vi "notes_load_xml.vi"(8 "error in":errorcluster, 10 "child node in":refnum<k20>) -> (0 "error out":errorcluster, 2 "child node out":refnum<k20>, 3 "notes":string)   [LabVIEW 2012]
doc: "Loads notes from xml file. Expected format for xml node passed in is:\n\n<Notes>%s</Notes>\n\nMTL 2013 Jan 1"
uses:
  <vilib>/xml/Close Reference(Node).vi
  <vilib>/xml/NI_XML.lvlib
  <resource>/objmgr/DOMUserDefRef.rc
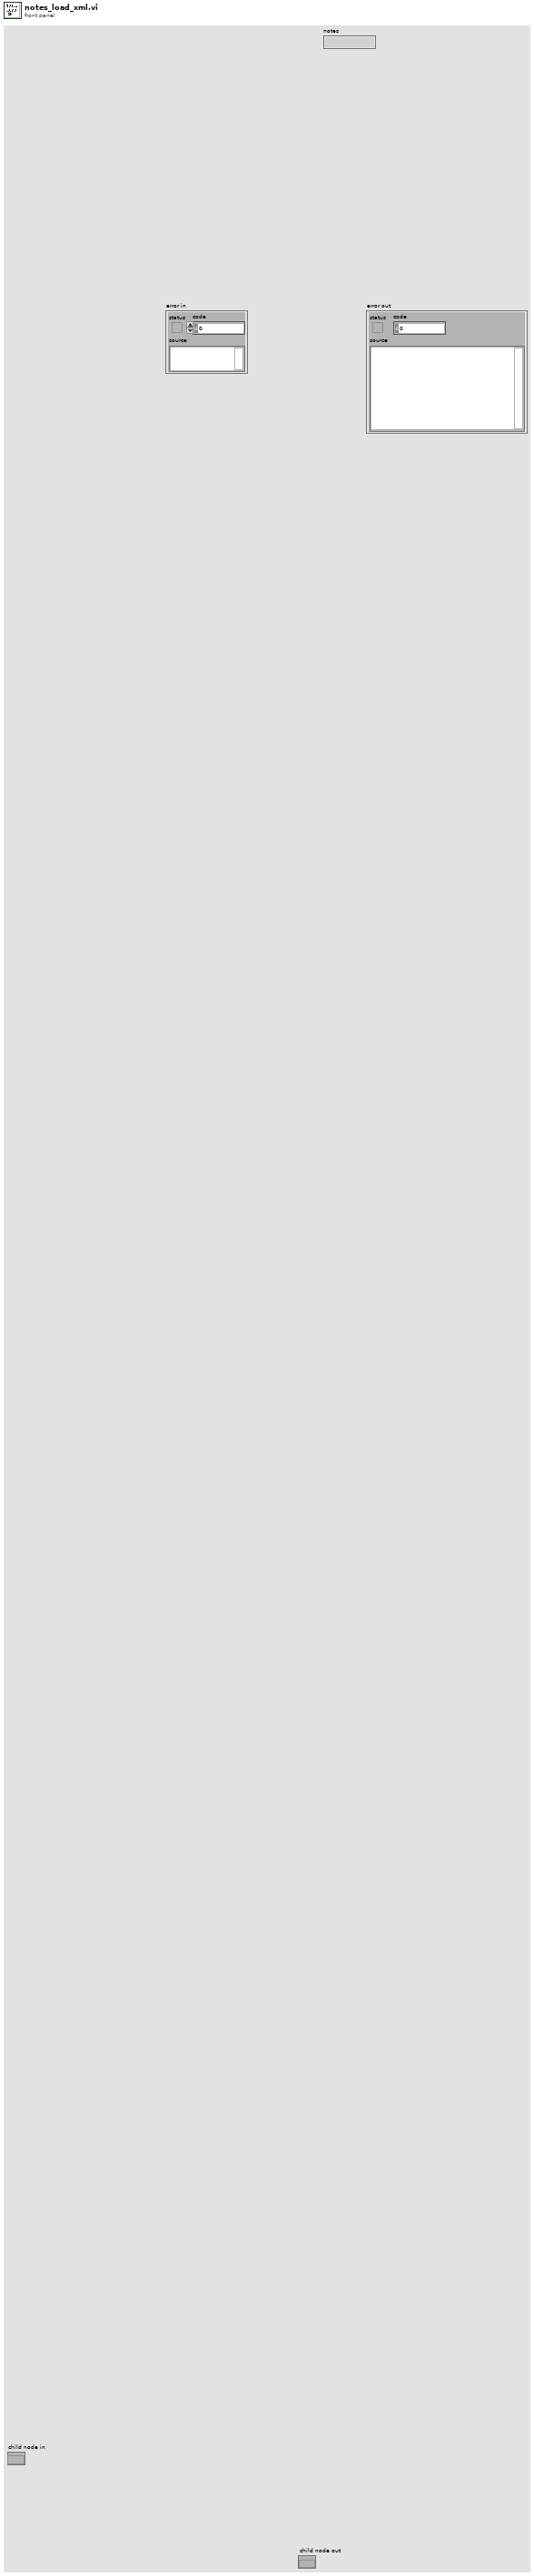
[diagram p1: front panel]
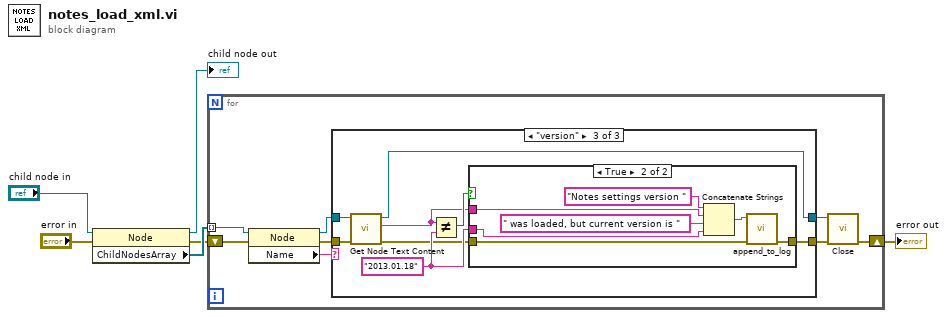
[diagram p0: block diagram]
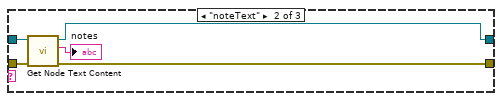
[diagram p3: hidden frame]
diagram:
  n1 = property class="Node"(reference="child node in", error in="error in") -> (reference out=→"child node out":refnum<k20>, error out=w2:errorcluster, "ChildNodesArray"=w4:refnum<k20>[])
  n2 = for {
    tunnel: w4 -> [w14] mode=indexing
    shift-right: [w12] -> w1
    shift-left: w2 -> [w13]
    n3 = property class="Node"(reference=w14, error in=w13) -> (reference out=w11:refnum<k20>, error out=w9:errorcluster, "Name"=w8:string)
    n4 = case shown="\"version\"" w8 {
      tunnel: w11 -> [w16 w18 w28]
      tunnel: [w15 w19 w23] -> w10
      tunnel: w9 -> [w15 w20 w29]
      tunnel: [w16 w17 w22] -> w7
      frame "None", Default {
      }
      frame "noteText" {
        n5 = call <vilib>:"Get Node Text Content.vi"("error in (no error)"=w20, "node in"=w18) -> ("error out"=w19:errorcluster, "node text"=→"notes":string, "node out"=w17:refnum<k20>)  [unwired: 7 in]
      }
      frame "version" {
        w25 = "2013.01.18" ("y")
        n6 = call <vilib>:"Get Node Text Content.vi"("error in (no error)"=w29, "node in"=w28) -> ("error out"=w24:errorcluster, "node text"=w26:string, "node out"=w22:refnum<k20>)  [unwired: 7 in]
        n7 = Not Equal?(x=w26, y=w25) -> (x != y?=w27:bool)
        n8 = case shown="True" w27 {
          tunnel: w26 -> [_ w36]
          tunnel: w25 -> [_ w34]
          tunnel: w24 -> [w30 w32]
          tunnel: [w30 w31] -> w23
          frame False {
          }
          frame True {
            n9 = Concatenate Strings("Notes settings version " ("string"), w36, " was loaded, but current version is " ("string"), w34) -> (w33:string)
            n10 = call "append_to_log.vi"("error in"=w32, "string"=w33) -> ("error out"=w31:errorcluster)  [unwired: 8 in, 1 out]
          }
        }
      }
    }
    n11 = call-poly <vilib>:"Close.vi"("error in (no error)"=w10, "node"=w7) -> ("error out"=w12:errorcluster)  [unwired: 7 in]
  }
  "error out" <- w1
